vi "Runner.ReadLinkerInfo.vi"(7 "Recursive?":bool, 8 "error in (no error)":errorcluster, 10 "VI Paths":path[](array[path]), 11 "Test Runner in":refnum<class "Test Runner.lvclass">) -> (0 "error out":errorcluster, 1 "Linker:Read Info From File":T2(array[cluster]), 2 "VI Paths (dup)":path[](array[path]), 3 "Test Runner out":refnum<class "Test Runner.lvclass">)   [LabVIEW 2013, in "Caraya.lvlib" / "Test Runner.lvclass"]
uses:
  Test Runner.lvclass
  <vilib>/Utility/lvfile.llb/LVFileType.ctl
  Test Runner.lvclass/Test Runner.ctl
  <vilib>/Utility/lvfile.llb/NI_FileType.lvlib
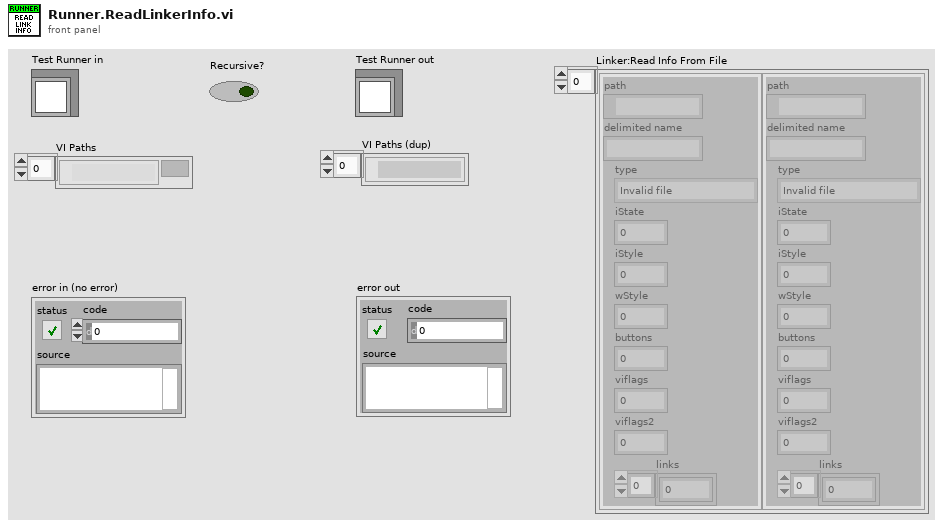
[diagram p1: front panel]
types:
  T1 = typedef "NI_FileType.lvlib/LVFileType.ctl" = enum32{"Invalid file", "Unknown type", "Instrument", "Control", "Polymorphic VI", "Project", "Library", "LVClass", "XControl", "XNode", "Shared library", ".NET assembly", "ActiveX interface", "CIN", "Run-time menu", "Palette menu", "Help file", "LLB", "XNode Edit Dependency", "Class Private Data Control", "Statechart", "MathScript .m file", "Ladder Diagram", "LVLibp", "XNode Build Dependency"}
  T2 = cluster{"path":path, "delimited name":string, "type":T1, "iState":u32, "iStyle":u16, "wStyle":u16, "buttons":u16, "viflags":u32, "viflags2":u32, "links":u32[]}[]
  T3 = typedef "NI_FileType.lvlib/LVFileType.ctl" = enum32{"Invalid file", "Unknown type", "Instrument", "Control", "Polymorphic VI", "Project", "Library", "LVClass", "XControl", "XNode", "Shared library", ".NET assembly", "ActiveX interface", "CIN", "Run-time menu", "Palette menu", "Help file", "LLB", "XNode Edit Dependency", "Class Private Data Control", "Statechart", "MathScript .m file", "Ladder Diagram", "LVLibp"}
  T4 = cluster{"path":path, "delimited name":string, "type":T3, "iState":u32, "iStyle":u16, "wStyle":u16, "buttons":u16, "viflags":u32, "viflags2":u32, "links":u32[]}[]
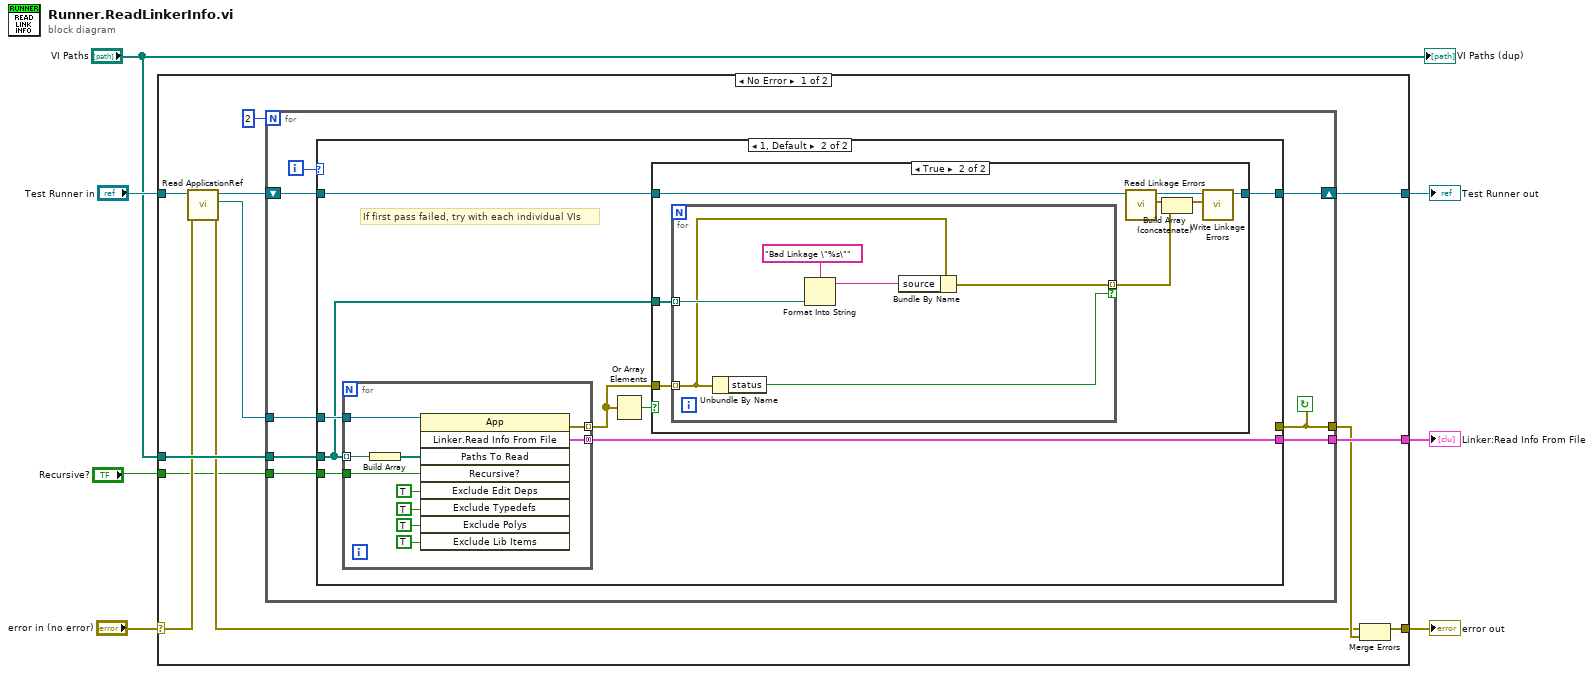
[diagram p0: block diagram]
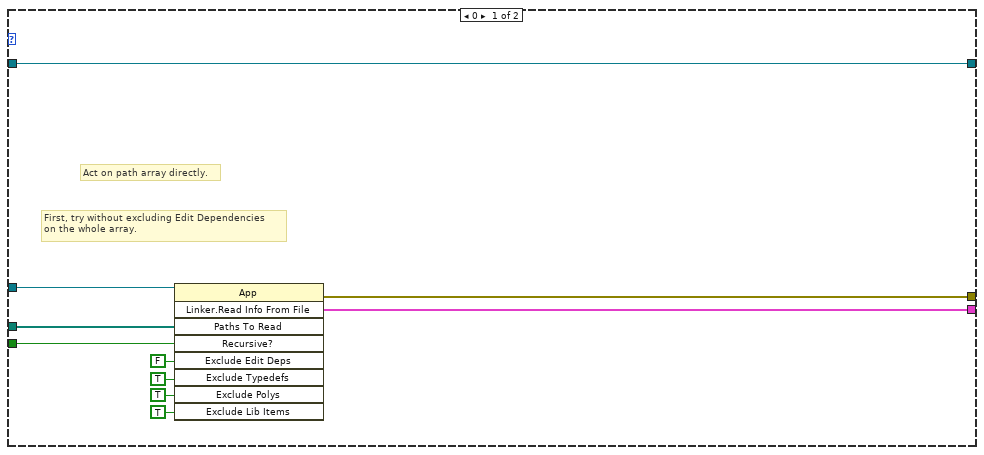
[diagram p2: hidden frame]
diagram:
  n1 = case shown="No Error" "error in (no error)" {
    selector: "error in (no error)" -> [w11 w72]
    tunnel: [w19 _] -> w7
    tunnel: [w15 w72] -> w6
    tunnel: [w17 w71] -> w5
    tunnel: "Test Runner in" -> [w13 w71]
    tunnel: "VI Paths" -> [w16 _]
    tunnel: "Recursive?" -> [w8 _]
    frame No Error {
      n2 = call "Read ApplicationRef.vi"("error in (no error)"=w11, "Test Runner in"=w13) -> ("error out"=w10:errorcluster, "Application"=w9:refnum<vi>, "Test Runner out"=w12:refnum<class "Test Runner.lvclass">)  [unwired: 7 in]
      n3 = for {
        N: 2 -> [_]
        tunnel: w16 -> [w27]
        tunnel: [w26] -> w19
        tunnel: [w24] -> w14
        shift-right: [w23] -> w17
        shift-left: w12 -> [w22]
        tunnel: w9 -> [w21]
        tunnel: w8 -> [w20]
        i -> [w25]
        stop <- w24 continue-if-true
        n4 = case shown="1, Default" w25 {
          tunnel: w27 -> [w33 w38]
          tunnel: [w32 w45] -> w26
          tunnel: [w31 _] -> w24
          tunnel: [w30 w42] -> w23
          tunnel: w22 -> [w30 w41]
          tunnel: w21 -> [w29 w40]
          tunnel: w20 -> [w28 w39]
          frame 0 {
            # "First, try without excluding Edit Dependencies\non the whole array."
            # "Act on path array directly."
            n5 = invoke class="App" method="Linker.Read Info From File"(reference=w29, "Paths To Read"=w33, "Recursive?"=w28, "Exclude Edit Deps"=FALSE ("Exclude Edit Time Dependencies"), "Exclude Typedefs"=TRUE, "Exclude Polys"=TRUE ("Exclude Poly VIs"), "Exclude Lib Items"=TRUE ("Exclude Unused Library Items")) -> (error out=w31:errorcluster, "Linker.Read Info From File"=w32:T4)  [unwired: 2 in, 7 out]
          }
          frame 1, Default {
            # "If first pass failed, try with each individual VIs"
            n6 = for {
              tunnel: w38 -> [w61] mode=indexing
              tunnel: [w66] -> w45 mode=concatenating
              tunnel: [w65] -> w43 mode=indexing
              tunnel: w40 -> [w63]
              tunnel: w39 -> [w62]
              n7 = Build Array(w61) -> (w64:path[])
              n8 = invoke class="App" method="Linker.Read Info From File"(reference=w63, "Paths To Read"=w64, "Recursive?"=w62, "Exclude Edit Deps"=TRUE ("Exclude Edit Time Dependencies"), "Exclude Typedefs"=TRUE, "Exclude Polys"=TRUE ("Exclude Poly VIs"), "Exclude Lib Items"=TRUE ("Exclude Unused Library Items")) -> (error out=w65:errorcluster, "Linker.Read Info From File"=w66:T4)  [unwired: 2 in, 7 out]
            }
            n9 = Or Array Elements(Boolean array=w43) -> (logical OR=w44:bool)
            n10 = case shown="True" w44 {
              tunnel: w43 -> [_ w54]
              tunnel: [w46 w51] -> w42
              tunnel: w41 -> [w46 w52]
              tunnel: w38 -> [_ w47]
              frame False {
              }
              frame True {
                n11 = for {
                  tunnel: w54 -> [w56] mode=indexing
                  tunnel: [w60] -> w49 mode=indexing if=w57
                  tunnel: w47 -> [w58] mode=indexing
                  n12 = Unbundle By Name(w56) -> ("status"=w57:bool)
                  n13 = Format Into String(format string="Bad Linkage \"%s\"", w58) -> (resulting string=w59:string)  [unwired: 2 in, 1 out]
                  n14 = Bundle By Name(cluster=w56, "source"=w59) -> (w60:errorcluster)
                }
                n15 = call "Read Linkage Errors.vi"("Test Runner in"=w52) -> ("Linkage Errors"=w50:errorcluster[], "Test Runner out"=w53:refnum<class "Test Runner.lvclass">)  [unwired: 8 in, 1 out]
                n16 = Build Array (concatenate)(w50, w49) -> (w48:errorcluster[])
                n17 = call "Write Linkage Errors.vi"("Linkage Errors"=w48, "Test Runner in"=w53) -> ("Test Runner out"=w51:refnum<class "Test Runner.lvclass">)  [unwired: 8 in, 1 out]
              }
            }
          }
        }
      }
      n18 = Merge Errors(w10, w14) -> (w15:errorcluster)
    }
    frame Error {
    }
  }
  "Linker:Read Info From File" <- w7
  "error out" <- w6
  "Test Runner out" <- w5
  "VI Paths (dup)" <- "VI Paths"
